vi "Maui 2.0.GetProcesses.vi"(8 "error in (no error)":errorcluster, 10 "Subpanels":refnum<class "SMO.lvclass">[](array[class])) -> (0 "error out":errorcluster, 2 "Processes":refnum<vi>[](array[refnum]))   [LabVIEW 2019, in "Maui 2.0.lvclass"]
uses:
  Maui 2.0.lvclass
  <vilib>/JKI/JKI SMO/SMO/SMO.lvclass
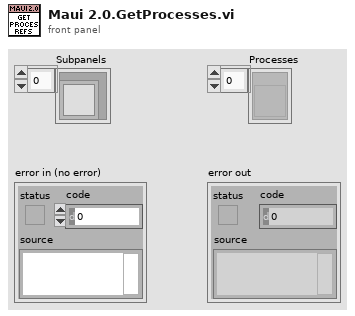
[diagram p1: front panel]
types:
  T1 = typedef "SMO.lvclass/RegisteredProcessData--Cluster.ctl" = cluster{"Name":string, "Static VI Ref":refnum<vi>, "Running":bool, "NotifierRef":u32}
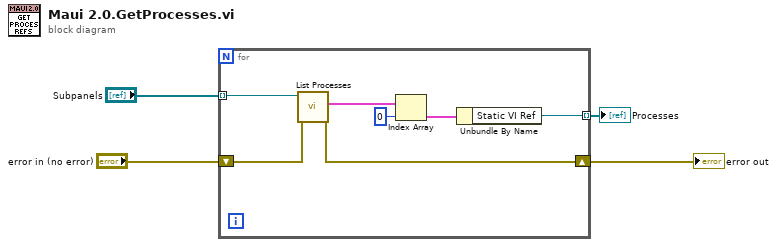
[diagram p0: block diagram]
diagram:
  n1 = for {
    tunnel: "Subpanels" -> [w11] mode=indexing
    shift-right: [w9] -> w2
    shift-left: "error in (no error)" -> [w10]
    tunnel: [w5] -> w1 mode=indexing
    n2 = call <vilib>:"List Processes.vi"("error in (no error)"=w10, "SMO"=w11) -> ("error out"=w9:errorcluster, "Registered Processes"=w8:T1[])  [unwired: 7 in, 1 out]
    n3 = Index Array(array=w8, index=0) -> (element=w6:T1)
    n4 = Unbundle By Name(w6) -> ("Static VI Ref"=w5:refnum<vi>)
  }
  "error out" <- w2
  "Processes" <- w1
